vi "Open File For Log.vi"(8 "Error In":errorcluster, 10 "File Path":path, 11 "FileLogger In":refnum<class "FileLogger.lvclass">) -> (0 "Error Out":errorcluster, 3 "FileLogger Out":refnum<class "FileLogger.lvclass">)   [LabVIEW 2019, in "FileLogger.lvclass"]
uses:
  FileLogger.lvclass
  FileLogger.lvclass/FileLogger.ctl
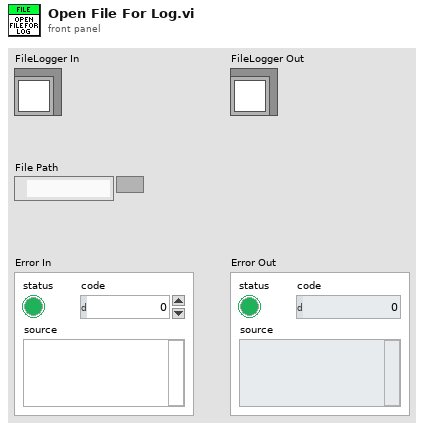
[diagram p1: front panel]
types:
  T1 = enum16{"open", "replace", "create", "open or create", "replace or create", "replace or create with confirmation"}
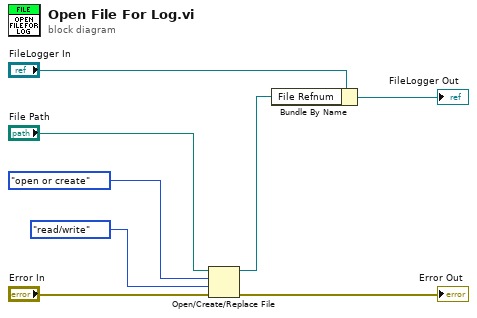
[diagram p0: block diagram]
diagram:
  n1 = Open/Create/Replace File(file path (use dialog)="File Path", error in="Error In", operation (0:open)=T1."open or create", access (0:read/write)=enum16{"read/write", "read-only", "write-only"}."read/write") -> (refnum out=w5:refnum<file>, error out=→"Error Out":errorcluster)  [unwired: 2 in, 1 out]
  n2 = Bundle By Name(cluster="FileLogger In", "File Refnum"=w5) -> (→"FileLogger Out":refnum<class "FileLogger.lvclass">)
